vi "Флаг рег..vi"(1 "Reset":bool, 2 "C":bool, 3 "Enter":T2) -> (0 "Exit":T1)   [LabVIEW 2017]
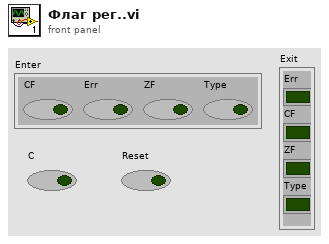
[diagram p1: front panel]
types:
  T1 = cluster{"Err":bool, "CF":bool, "ZF":bool, "Type":bool}
  T2 = cluster{"CF":bool, "Err":bool, "ZF":bool, "Type":bool}
  T3 = cluster{"cf":bool, "zf":bool, "err":bool, "type":bool}
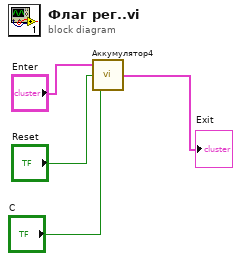
[diagram p0: block diagram]
diagram:
  n1 = call "Аккумулятор4.vi"("Reset"="C", "C"="Reset", "Enter"="Enter") -> ("Exit"=→"Exit":T3)
